vi "Apply linear and non linear zoom on image and pixel maps based on system type (Galvo-Reso).vi"(4 "Y Pixel Map IN":i32[](array[numeric]), 6 "X Pixel Map IN":i32[](array[numeric]), 7 "Non-Linear X Component (array of 1's for Galvo)":dbl[](array[numeric]), 9 "Y Linear Zoom (0.5 or 3)":dbl, 10 "X Linear Zoom (0.5 or 3)":dbl, 11 "Image Ref IN":T1) -> (1 "Y Pixel map OUT":i32[](array[numeric]), 2 "X Pixel map OUT":i32[](array[numeric]), 3 "Image Ref OUT":T1)   [LabVIEW 2012]
uses:
  <vilib>/vision/Image Controls.llb/IMAQ Image.ctl
  <vilib>/vision/NI_Vision_Development_Module.lvlib
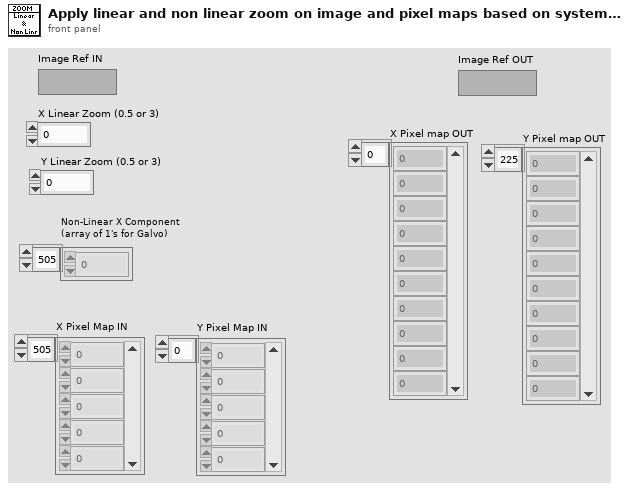
[diagram p1: front panel]
types:
  T1 = typedef "IMAQ Image.ctl" = refnum<image>
  T2 = typedef "Image Type" = u32
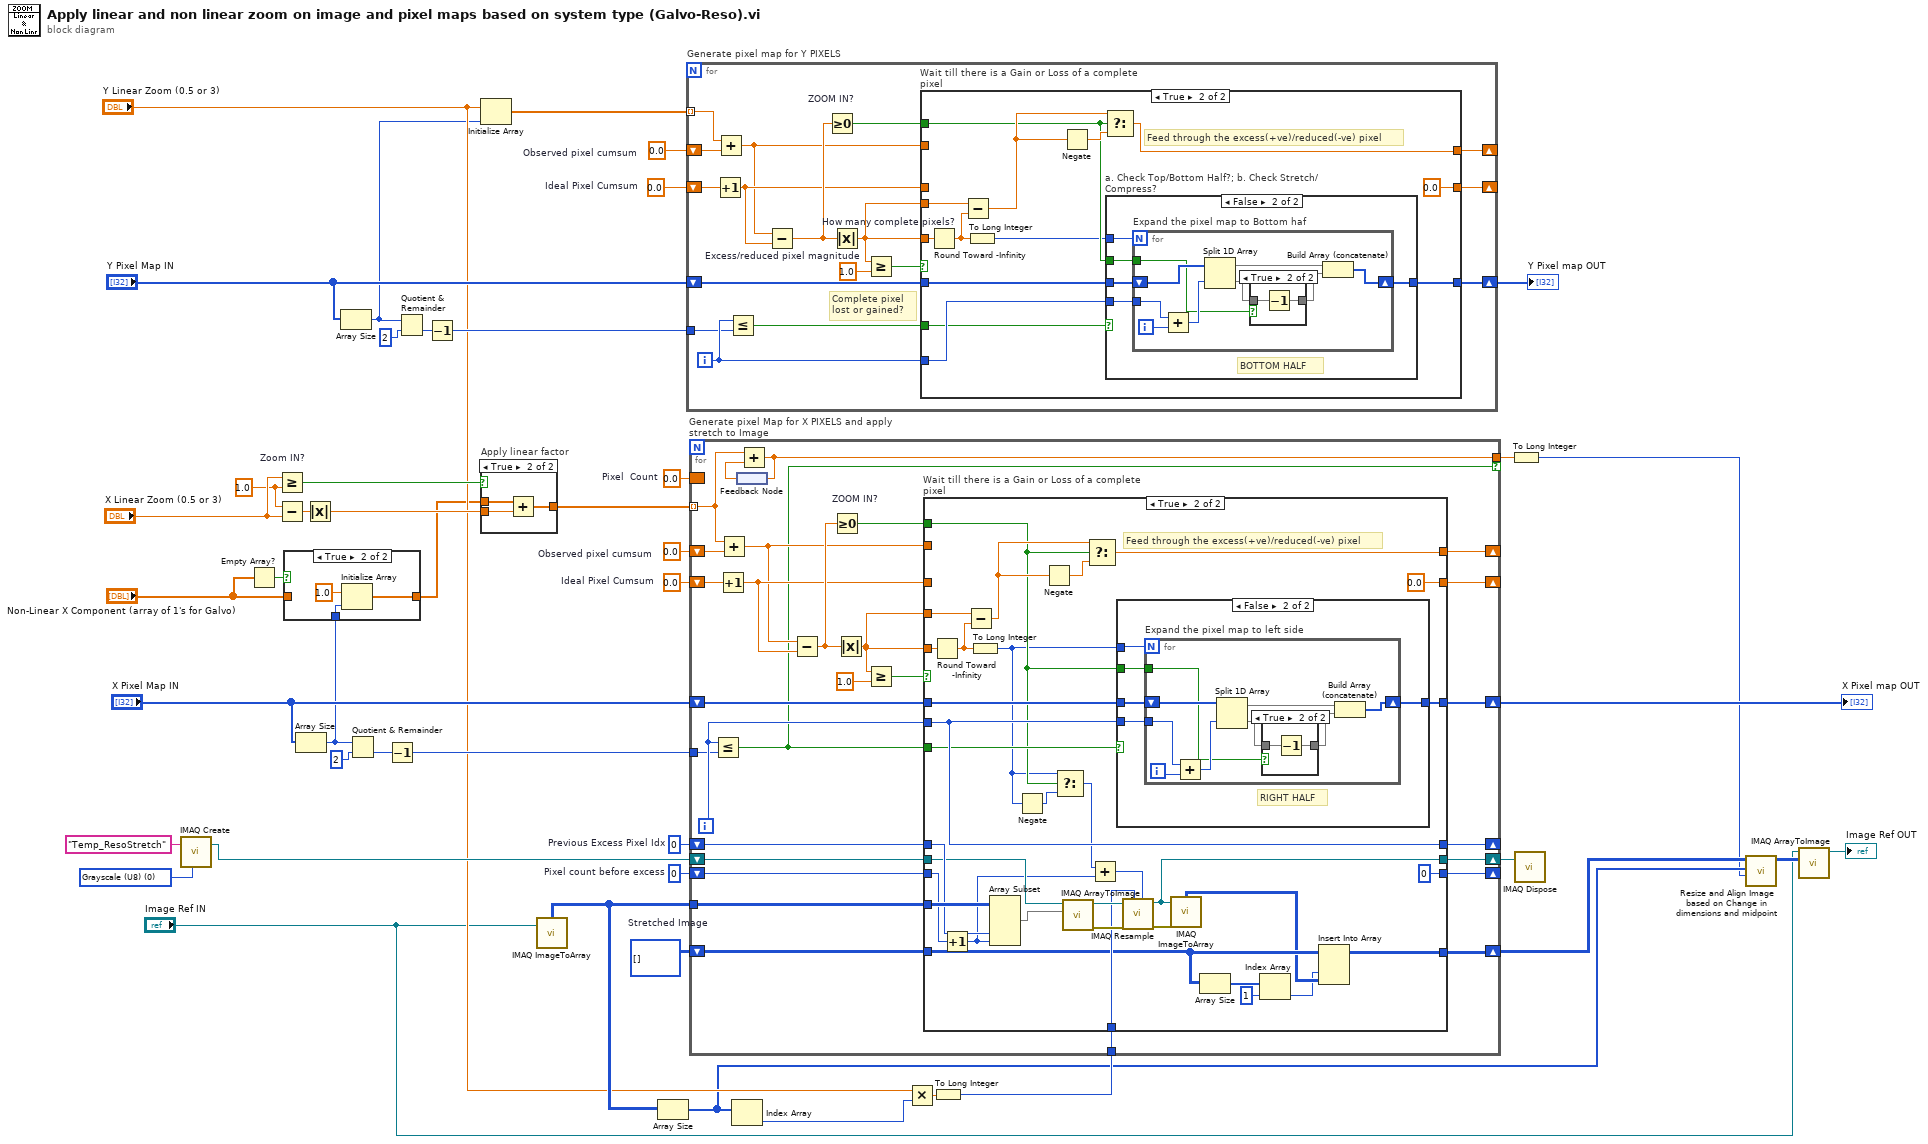
[diagram p0: block diagram]
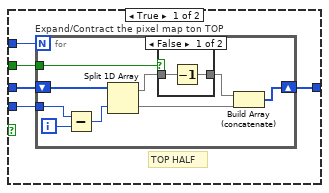
[diagram p4: hidden frame]
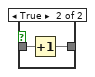
[diagram p5: hidden frame]
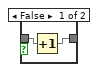
[diagram p6: hidden frame]
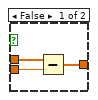
[diagram p7: hidden frame]
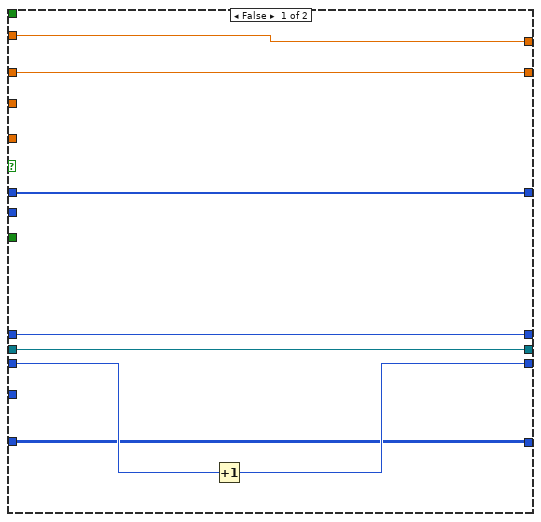
[diagram p8: hidden frame]
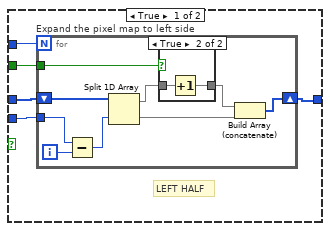
[diagram p9: hidden frame]
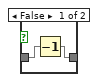
[diagram p10: hidden frame]
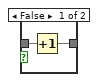
[diagram p11: hidden frame]
diagram:
  w20 = 0.0  # Observed pixel cumsum
  w19 = 0.0  # Ideal Pixel Cumsum
  w7 = 0.0  # Pixel  Count
  w28 = u8[][] []  # Stretched Image
  w31 = T2 0 items=["Grayscale (U8)", "Grayscale (I16)", "Grayscale (SGL)", "Complex (CSG)", "RGB (U32)", "HSL (U32)", "RGB (U64)", "Grayscale (U16)"] ("Image Type")
  w33 = 0  # Pixel count before excess
  w34 = 0  # Previous Excess Pixel Idx
  w42 = 0.0  # Observed pixel cumsum
  w43 = 0.0  # Ideal Pixel Cumsum
  w39 = 1.0 ("y")
  n1 = call "IMAQ Create"("Image Name"="Temp_ResoStretch", "Image Type"=w31) -> ("New Image"=w29:T1)  [unwired: 3 in, 1 out]
  n2 = Empty Array?(array="Non-Linear X Component (array of 1's for Galvo)") -> (empty?=w11:bool)
  n3 = Greater Or Equal? "Zoom IN?"(x="X Linear Zoom (0.5 or 3)", y=w39) -> (x >= y?=w38:bool)
  n4 = Subtract(x=w39, y="X Linear Zoom (0.5 or 3)") -> (x-y=w46:dbl)
  n5 = Array Size(array="X Pixel Map IN") -> (size(s)=w8:i32)
  n6 = case shown="True" w11 {
    tunnel: "Non-Linear X Component (array of 1's for Galvo)" -> [w47 _]
    tunnel: [w47 w48] -> w9
    tunnel: w8 -> [_ w49]
    frame False {
    }
    frame True {
      n7 = Initialize Array(1.0 ("element"), w49) -> (w48:dbl[])
    }
  }
  n8 = Absolute Value(x=w46) -> (abs(x)=w40:dbl)
  n9 = Array Size(array="Y Pixel Map IN") -> (size(s)=w14:i32)
  n10 = Quotient & Remainder(x=w8, y=2) -> (floor(x/y)=w36:i32)  [unwired: 1 out]
  n11 = Decrement(x=w36) -> (x-1=w24:i32)
  n12 = Quotient & Remainder(x=w14, y=2) -> (floor(x/y)=w17:i32)  [unwired: 1 out]
  n13 = Decrement(x=w17) -> (x-1=w21:i32)
  n14 = Initialize Array("Y Linear Zoom (0.5 or 3)", w14) -> (w13:dbl[])
  n15 = case "Apply linear factor" shown="True" w38 {
    tunnel: w9 -> [w53 w56]
    tunnel: [w52 w55] -> w44
    tunnel: w40 -> [w51 w54]
    frame False {
      n16 = Subtract(x=w53, y=w51) -> (x-y=w52:dbl[])
    }
    frame True {
      n17 = Add(x=w56, y=w54) -> (x+y=w55:dbl[])
    }
  }
  n18 = call "IMAQ ImageToArray"("Image"="Image Ref IN") -> ("Image Pixels (U8)"=w30:u8[][])  [unwired: 3 in, 4 out]
  n19 = Array Size(array=w30) -> (size(s)=w5:i32[])
  n20 = for "Generate pixel map for Y PIXELS" {
    tunnel: w13 -> [w60] mode=indexing
    shift-right: [w67] -> _
    shift-left: w20 -> [w65]
    shift-right: [w68] -> _
    shift-left: w19 -> [w73]
    tunnel: w21 -> [w58]
    shift-right: [w62] -> w12
    shift-left: "Y Pixel Map IN" -> [w64]
    i -> [w59]
    # "Complete pixel lost or gained?"
    n21 = Increment(x=w73) -> (x+1=w69:dbl)
    n22 = Add(x=w60, y=w65) -> (x+y=w66:dbl)
    n23 = Less Or Equal?(x=w59, y=w58) -> (x <= y?=w57:bool)
    n24 = Subtract "Excess/reduced pixel magnitude"(x=w66, y=w69) -> (x-y=w70:dbl)
    n25 = Greater Or Equal To 0? "ZOOM IN?"(x=w70) -> (x >= 0?=w63:bool)
    n26 = Absolute Value(x=w70) -> (abs(x)=w61:dbl)
    n27 = Greater Or Equal?(x=w61, y=1.0) -> (x >= y?=w71:bool)
    n28 = case "Wait till there is a Gain or Loss of a complete pixel" shown="True" w71 {
      tunnel: w61 -> [_ w85]
      tunnel: w69 -> [w76 _]
      tunnel: [w76 0.0] -> w68
      tunnel: [w75 w81] -> w67
      tunnel: w66 -> [w75 _]
      tunnel: w64 -> [w74 w88]
      tunnel: w59 -> [_ w80]
      tunnel: w63 -> [_ w78]
      tunnel: w61 -> [_ w87]
      tunnel: [w74 w86] -> w62
      tunnel: w57 -> [_ w79]
      frame False {
      }
      frame True {
        # "Feed through the excess(+ve)/reduced(-ve) pixel"
        n29 = Round Toward -Infinity "How many complete pixels?"(1:w87) -> (0:w84:dbl)
        n30 = Subtract(x=w85, y=w84) -> (x-y=w83:dbl)
        n31 = To Long Integer(number=w84) -> (32bit integer=w77:i32)
        n32 = Negate(x=w83) -> (-x=w82:dbl)
        n33 = Select(t=w83, s=w78, f=w82) -> (s? t:f=w81:dbl)
        n34 = case "a. Check Top/Bottom Half?; b. Check Stretch/Compress?" shown="False" w79 {
          tunnel: w88 -> [w94 w112]
          tunnel: w78 -> [w90 w108]
          tunnel: w80 -> [w93 w111]
          tunnel: w77 -> [w92 w110]
          tunnel: [w91 w109] -> w86
          frame True {
            # "TOP HALF"
            n35 = for "Expand/Contract the pixel map ton TOP" {
              N: w92 -> [_]
              tunnel: w93 -> [w98]
              shift-right: [w96] -> w91
              shift-left: w94 -> [w103]
              tunnel: w90 -> [w95]
              i -> [w99]
              n36 = Subtract(x=w98, y=w99) -> (x-y=w97:i32)
              n37 = Split 1D Array(array=w103, index=w97) -> (first subarray=w102:i32[], second subarray=w100:i32[])
              n38 = case shown="False" w95 {
                tunnel: w102 -> [w105 w107]
                tunnel: [w104 w106] -> w101
                frame False {
                  n39 = Decrement(x=w105) -> (x-1=w104:i32[])
                }
                frame True {
                  n40 = Increment(x=w107) -> (x+1=w106:i32[])
                }
              }
              n41 = Build Array (concatenate)(w101, w100) -> (w96:i32[])
            }
          }
          frame False {
            # "BOTTOM HALF"
            n42 = for "Expand the pixel map to Bottom haf" {
              N: w110 -> [_]
              tunnel: w111 -> [w119]
              shift-right: [w117] -> w109
              shift-left: w112 -> [w121]
              tunnel: w108 -> [w116]
              i -> [w120]
              n43 = Add(x=w119, y=w120) -> (x+y=w118:i32)
              n44 = Split 1D Array(array=w121, index=w118) -> (first subarray=w113:i32[], second subarray=w115:i32[])
              n45 = case shown="True" w116 {
                tunnel: w115 -> [w123 w125]
                tunnel: [w122 w124] -> w114
                frame False {
                  n46 = Increment(x=w123) -> (x+1=w122:i32[])
                }
                frame True {
                  n47 = Decrement(x=w125) -> (x-1=w124:i32[])
                }
              }
              n48 = Build Array (concatenate)(w113, w114) -> (w117:i32[])
            }
          }
        }
      }
    }
  }
  "Y Pixel map OUT" <- w12
  n49 = Index Array(array=w5) -> (element=w23:i32)  [unwired: 1 in]
  n50 = Multiply(x="Y Linear Zoom (0.5 or 3)", y=w23) -> (x*y=w27:dbl)
  n51 = To Long Integer(number=w27) -> (32bit integer=w26:i32)
  n52 = for "Generate pixel Map for X PIXELS and apply stretch to Image" {
    tunnel: w44 -> [w128] mode=indexing
    shift-right: [w148] -> _
    shift-left: w42 -> [w146]
    shift-right: [w149] -> _
    shift-left: w43 -> [w154]
    tunnel: w24 -> [w131]
    shift-right: [w143] -> w37
    shift-left: "X Pixel Map IN" -> [w145]
    tunnel: w30 -> [w141]
    shift-right: [w140] -> _
    shift-left: w34 -> [w139]
    shift-right: [w137] -> _
    shift-left: w33 -> [w138]
    tunnel: w26 -> [w135]
    shift-right: [w133] -> w6
    shift-left: w28 -> [w134]
    tunnel: [w127] -> w22 if=w130
    border: w7 -> [_]
    shift-right: [w126] -> w2
    shift-left: w29 -> [w136]
    i -> [w132]
    n53 = Less Or Equal?(x=w132, y=w131) -> (x <= y?=w130:bool)
    n54 = Increment(x=w154) -> (x+1=w150:dbl)
    n55 = Add(x=w128, y=w146) -> (x+y=w147:dbl)
    n56 = feedback #1() -> (w129:dbl)
    n57 = Add(x=w128, y=w129) -> (x+y=w127:dbl)
    n58 = feedback-in #1(w127) -> ()
    n59 = Subtract(x=w147, y=w150) -> (x-y=w151:dbl)
    n60 = Greater Or Equal To 0? "ZOOM IN?"(x=w151) -> (x >= 0?=w144:bool)
    n61 = Absolute Value(x=w151) -> (abs(x)=w142:dbl)
    n62 = Greater Or Equal?(x=w142, y=1.0) -> (x >= y?=w152:bool)
    n63 = case "Wait till there is a Gain or Loss of a complete pixel" shown="True" w152 {
      tunnel: w142 -> [_ w192]
      tunnel: w150 -> [w162 _]
      tunnel: [w162 0.0] -> w149
      tunnel: [w161 w188] -> w148
      tunnel: w147 -> [w161 _]
      tunnel: w145 -> [w160 w195]
      tunnel: w132 -> [_ w186]
      tunnel: w144 -> [_ w167]
      tunnel: w142 -> [_ w194]
      tunnel: [w160 w193] -> w143
      tunnel: w141 -> [_ w187]
      tunnel: [w157 w186] -> w140
      tunnel: w139 -> [w157 w185]
      tunnel: w138 -> [w159 w184]
      tunnel: [w158 0] -> w137
      tunnel: w136 -> [w155 w182]
      tunnel: w135 -> [_ w179]
      tunnel: w134 -> [w156 w173]
      tunnel: [w156 w170] -> w133
      tunnel: w130 -> [_ w171]
      tunnel: [w155 w163] -> w126
      frame False {
        n64 = Increment(x=w159) -> (x+1=w158:i32)
      }
      frame True {
        # "Feed through the excess(+ve)/reduced(-ve) pixel"
        n65 = Round Toward -Infinity(1:w194) -> (0:w191:dbl)
        n66 = Increment(x=w184) -> (x+1=w178:i32)
        n67 = Subtract(x=w192, y=w191) -> (x-y=w190:dbl)
        n68 = To Long Integer(number=w191) -> (32bit integer=w165:i32)
        n69 = Array Subset(array=w187, index (col)=w185, length (col)=w178) -> (w168:u8[][])  [unwired: 2 in]
        n70 = Negate(x=w165) -> (-x=w166:i32)
        n71 = Negate(x=w190) -> (-x=w189:dbl)
        n72 = Select(t=w165, s=w167, f=w166) -> (s? t:f=w164:i32)
        n73 = call "IMAQ ArrayToImage"("Image Pixels (U8)"=w168, "Image"=w182) -> ("error out"=w181:errorcluster, "Image Out"=w180:T1)  [unwired: 8 in]
        n74 = Select(t=w190, s=w167, f=w189) -> (s? t:f=w188:dbl)
        n75 = Add(x=w164, y=w178) -> (x+y=w177:i32)
        n76 = case shown="False" w171 {
          tunnel: w195 -> [w201 w219]
          tunnel: w167 -> [w197 w215]
          tunnel: w186 -> [w200 w218]
          tunnel: w165 -> [w199 w217]
          tunnel: [w198 w216] -> w193
          frame True {
            # "LEFT HALF"
            n77 = for "Expand the pixel map to left side" {
              N: w199 -> [_]
              tunnel: w200 -> [w205]
              shift-right: [w203] -> w198
              shift-left: w201 -> [w210]
              tunnel: w197 -> [w202]
              i -> [w206]
              n78 = Subtract(x=w205, y=w206) -> (x-y=w204:i32)
              n79 = Split 1D Array(array=w210, index=w204) -> (first subarray=w209:i32[], second subarray=w207:i32[])
              n80 = case shown="True" w202 {
                tunnel: w209 -> [w212 w214]
                tunnel: [w211 w213] -> w208
                frame False {
                  n81 = Decrement(x=w212) -> (x-1=w211:i32[])
                }
                frame True {
                  n82 = Increment(x=w214) -> (x+1=w213:i32[])
                }
              }
              n83 = Build Array (concatenate)(w208, w207) -> (w203:i32[])
            }
          }
          frame False {
            # "RIGHT HALF"
            n84 = for "Expand the pixel map to left side" {
              N: w217 -> [_]
              tunnel: w218 -> [w226]
              shift-right: [w224] -> w216
              shift-left: w219 -> [w228]
              tunnel: w215 -> [w223]
              i -> [w227]
              n85 = Add(x=w226, y=w227) -> (x+y=w225:i32)
              n86 = Split 1D Array(array=w228, index=w225) -> (first subarray=w220:i32[], second subarray=w222:i32[])
              n87 = case shown="True" w223 {
                tunnel: w222 -> [w230 w232]
                tunnel: [w229 w231] -> w221
                frame False {
                  n88 = Increment(x=w230) -> (x+1=w229:i32[])
                }
                frame True {
                  n89 = Decrement(x=w232) -> (x-1=w231:i32[])
                }
              }
              n90 = Build Array (concatenate)(w220, w221) -> (w224:i32[])
            }
          }
        }
        n91 = call "IMAQ Resample"("X Resolution"=w177, "Y Resolution"=w179, "error in (no error)"=w181, "Image Src"=w180) -> ("error out"=w176:errorcluster, "Image Dst Out"=w163:T1)  [unwired: 6 in]
        n92 = call "IMAQ ImageToArray"("error in (no error)"=w176, "Image"=w163) -> ("Image Pixels (U8)"=w172:u8[][])  [unwired: 2 in, 4 out]
        n93 = Array Size(array=w173) -> (size(s)=w174:i32[])
        n94 = Index Array(array=w174, index=1) -> (element=w169:i32)
        n95 = Insert Into Array(array=w173, index (col)=w169, new element=w172) -> (w170:u8[][])  [unwired: 1 in]
      }
    }
  }
  "X Pixel map OUT" <- w37
  n96 = To Long Integer(number=w22) -> (32bit integer=w4:i32)
  n97 = call "IMAQ Dispose"("Image"=w2) -> ()  [unwired: 5 in, 1 out]
  n98 = call "Resize and Align Image based on Change in dimensions and midpoint.vi"("Modified X Mid point Pixel (After Non-Linear Stretch)"=w4, "Initial Dimension (1D Array: Ypxls,XPxls)"=w5, "Modified Image Array (2D)"=w6) -> ("Resized-Recentered Image Array (2D)"=w3:u8[][])  [unwired: 8 in]
  n99 = call "IMAQ ArrayToImage"("Image Pixels (U8)"=w3, "Image"="Image Ref IN") -> ("Image Out"=→"Image Ref OUT":T1)  [unwired: 8 in, 1 out]
